vi "Calculate Blend Angles.vi"(11 "WayPoints":cluster{"x":dbl, "y":dbl, "th":dbl}[](array[cluster])) -> (2 "Waypoints out":cluster{"x":dbl, "y":dbl, "th":dbl}[](array[cluster]), 3 "Angles":dbl[](array[numeric]))   [LabVIEW 2018]
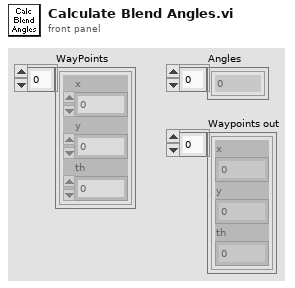
[diagram p1: front panel]
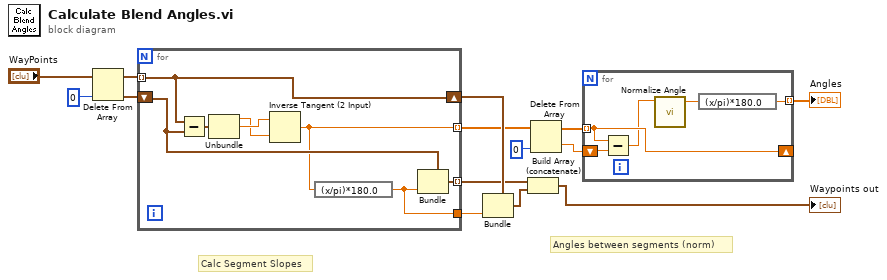
[diagram p0: block diagram]
diagram:
  # "Angles between segments (norm)"
  # "Calc Segment Slopes"
  n1 = Delete From Array(array="WayPoints", index=0) -> (deleted portion=w3:cluster{"x":dbl, "y":dbl, "th":dbl}, array with subset deleted=w4:cluster{"x":dbl, "y":dbl, "th":dbl}[])  [unwired: 1 in]
  n2 = for {
    shift-right: [w22] -> w10
    shift-left: w3 -> [w18]
    tunnel: w4 -> [w22] mode=indexing
    tunnel: [w17] -> w6 mode=indexing
    tunnel: [w16] -> w9 mode=indexing
    tunnel: [w15] -> w11
    n3 = Subtract(x=w22, y=w18) -> (x-y=w21:cluster{"x":dbl, "y":dbl, "th":dbl})
    n4 = Unbundle(w21) -> ("x"=w19:dbl, "y"=w20:dbl)  [unwired: 1 out]
    n5 = Inverse Tangent (2 Input)(1:w19, 2:w20) -> (0:w17:dbl)
    n6 = expression code="(x/pi)*180.0" ("radians to degrees")(w17) -> (w15:dbl)
    n7 = Bundle(cluster=w18, "th"=w15) -> (w16:cluster{"x":dbl, "y":dbl, "th":dbl})  [unwired: 2 in]
  }
  n8 = Bundle(cluster=w10, "th"=w11) -> (w12:cluster{"x":dbl, "y":dbl, "th":dbl})  [unwired: 2 in]
  n9 = Build Array (concatenate)(w9, w12) -> (→"Waypoints out":cluster{"x":dbl, "y":dbl, "th":dbl}[])
  n10 = Delete From Array(array=w6, index=0) -> (deleted portion=w8:dbl, array with subset deleted=w7:dbl[])  [unwired: 1 in]
  n11 = for {
    tunnel: w7 -> [w26] mode=indexing
    shift-right: [w26] -> _
    shift-left: w8 -> [w27]
    tunnel: [w23] -> w13 mode=indexing
    n12 = Subtract(x=w26, y=w27) -> (x-y=w25:dbl)
    n13 = call "Normalize Angle.vi"("Angle in r"=w25) -> ("Angle out r"=w24:dbl)  [unwired: 10 in]
    n14 = expression code="(x/pi)*180.0" ("radians to degrees")(w24) -> (w23:dbl)
  }
  "Angles" <- w13
